vi "Initialize.vi"(7 "Channel Name":string="Setpoint.ch%d.SP", 8 "error in":errorcluster, 9 "Number of Channels":u32=1, 10 "Instance Name":string, 11 "Control Mode in":refnum<class "Control Mode.lvclass">) -> (0 "error out":errorcluster, 2 "Channel":T1[](array[typedef]), 3 "Control Mode out":refnum<class "Control Mode.lvclass">)   [LabVIEW 2023, in "Control Mode.lvclass"]
uses:
  Control Mode.lvclass
  <vilib>/ADAS Replay HIL/Channels/Tag Wrapper/Tag Wrapper.lvlib
  Utilities/Utilities.lvlib
  <vilib>/ADAS Replay HIL/Channels/Tag Wrapper/Polymorphic/Open Consumer Tag (U16).vi
  <vilib>/ADAS Replay HIL/Channels/Tag Wrapper/Polymorphic/Set Default Value (U16).vi
  <vilib>/ADAS Replay HIL/Channels/Tag Wrapper/Polymorphic/Open Producer Tag (U16).vi
  Utilities/Channel.ctl
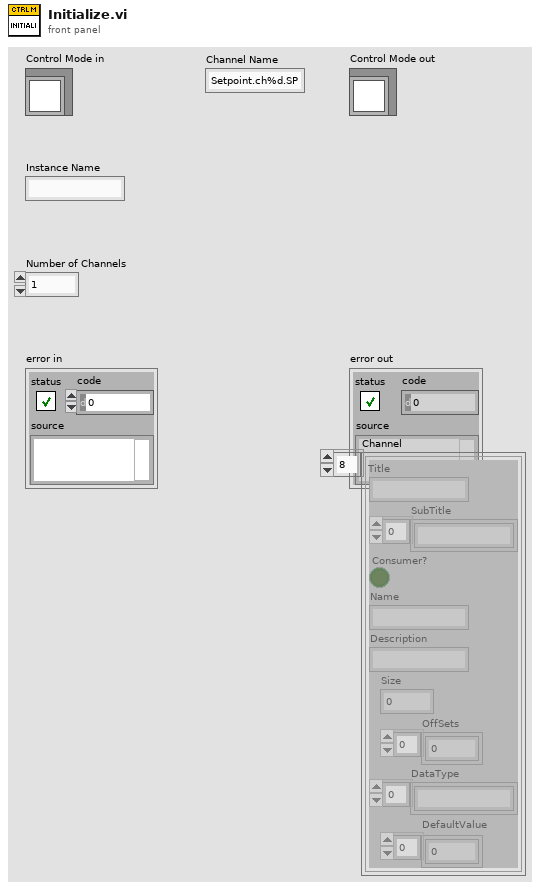
[diagram p1: front panel]
types:
  T1 = typedef "Utilities.lvlib/Channel.ctl" = cluster{"Title":string, "SubTitle":string[], "Consumer?":bool, "Name":string, "Description":string, "Size":i32, "OffSets":i32[], "DataType":string[], "DefaultValue":dbl[]}
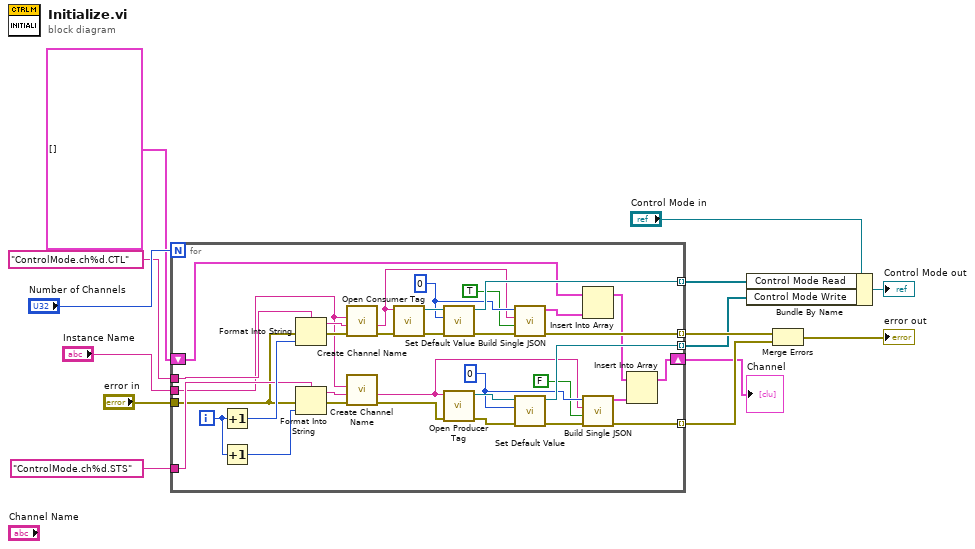
[diagram p0: block diagram]
diagram:
  n1 = for {
    N: "Number of Channels" -> [_]
    tunnel: "ControlMode.ch%d.CTL" ("ChannelName") -> [w47]
    tunnel: "error in" -> [w31]
    tunnel: [w20] -> w4 mode=indexing
    tunnel: [w22] -> w5 mode=indexing
    tunnel: "ControlMode.ch%d.STS" ("ChannelName") -> [w38]
    tunnel: [w36] -> w12 mode=indexing
    tunnel: [w35] -> w3 mode=indexing
    tunnel: "Instance Name" -> [w30]
    shift-right: [w16] -> w2
    shift-left: T1[] [] -> [w15]
    i -> [w39]
    w29 = u16 0 ("Default Value")
    w28 = u16 0 ("Default Value")
    n2 = Increment(x=w39) -> (x+1=w48:i32)
    n3 = Increment(x=w39) -> (x+1=w40:i32)
    n4 = Format Into String(format string=w47, error in=w31, w48) -> (resulting string=w46:string, error out=w33:errorcluster)  [unwired: 1 in]
    n5 = Format Into String(format string=w38, error in=w31, w40) -> (resulting string=w37:string, error out=w32:errorcluster)  [unwired: 1 in]
    n6 = call "Create Channel Name.vi"("error in"=w33, "Channel Name"=w46, "Plugin Name"=w30) -> ("error out"=w34:errorcluster, "Data Channel Name"=w27:string)  [unwired: 7 in]
    n7 = call "Create Channel Name.vi"("error in"=w32, "Channel Name"=w37, "Plugin Name"=w30) -> ("error out"=w42:errorcluster, "Data Channel Name"=w26:string)  [unwired: 7 in]
    n8 = call-poly <vilib>:"Open Consumer Tag.vi"("error in"=w34, "Channel Name"=w27) -> ("error out"=w44:errorcluster, "ADAS HIL Channel"=w45:refnum<k21>)  [unwired: 8 in]
    n9 = call-poly <vilib>:"Set Default Value.vi"("error in"=w44, "Default Value"=w28, "ADAS HIL Channel in"=w45) -> ("error out"=w21:errorcluster, "ADAS HIL Channel out"=w36:refnum<k21>)  [unwired: 7 in]
    n10 = call-poly <vilib>:"Open Producer Tag.vi"("error in"=w42, "Channel Name"=w26) -> ("error out"=w41:errorcluster, "ADAS HIL Channel"=w43:refnum<k21>)  [unwired: 8 in]
    n11 = call "Build Single JSON.vi"("error in"=w21, "Consumer?"=TRUE, "ChannelName"=w27, "Single"=w28) -> ("error out"=w20:errorcluster, "Channel"=w18:T1)  [unwired: 6 in]
    n12 = call-poly <vilib>:"Set Default Value.vi"("error in"=w41, "Default Value"=w29, "ADAS HIL Channel in"=w43) -> ("error out"=w23:errorcluster, "ADAS HIL Channel out"=w35:refnum<k21>)  [unwired: 7 in]
    n13 = Insert Into Array(array=w15, new element=w18) -> (w19:T1[])  [unwired: 1 in]
    n14 = call "Build Single JSON.vi"("error in"=w23, "Consumer?"=FALSE, "ChannelName"=w26, "Single"=w29) -> ("error out"=w22:errorcluster, "Channel"=w17:T1)  [unwired: 6 in]
    n15 = Insert Into Array(array=w19, new element=w17) -> (w16:T1[])  [unwired: 1 in]
  }
  "Channel" <- w2
  n16 = Bundle By Name(cluster="Control Mode in", "Control Mode Read"=w12, "Control Mode Write"=w3) -> (→"Control Mode out":refnum<class "Control Mode.lvclass">)
  n17 = Merge Errors(w4, w5) -> (→"error out":errorcluster)
